vi "mav_connection_write.vi"(8 "error in":errorcluster, 9 "Connection Type":enum32{"TCP", "SERIAL", "UDP"}(tab), 10 "data in":string, 11 "mav_connection_in":T2) -> (0 "error out":errorcluster, 3 "mav_connection_out":T1)   [LabVIEW 2023]
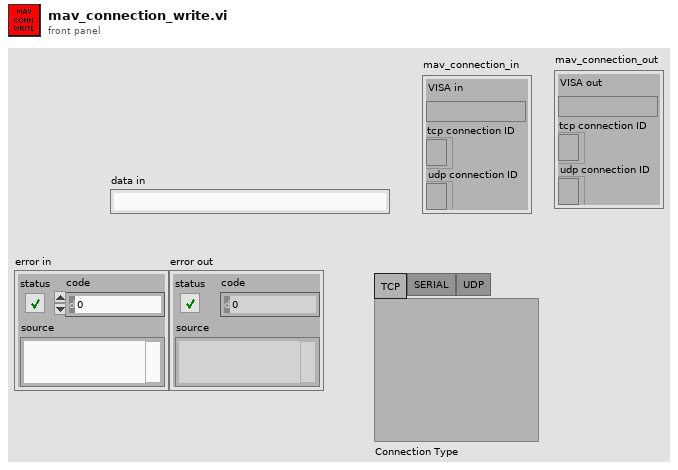
[diagram p1: front panel]
types:
  T1 = cluster{"VISA out":refnum<visa-resource-name>, "tcp connection ID":refnum<k5>, "udp connection ID":refnum<k16>}
  T2 = cluster{"VISA in":refnum<visa-resource-name>, "tcp connection ID":refnum<k5>, "udp connection ID":refnum<k16>}
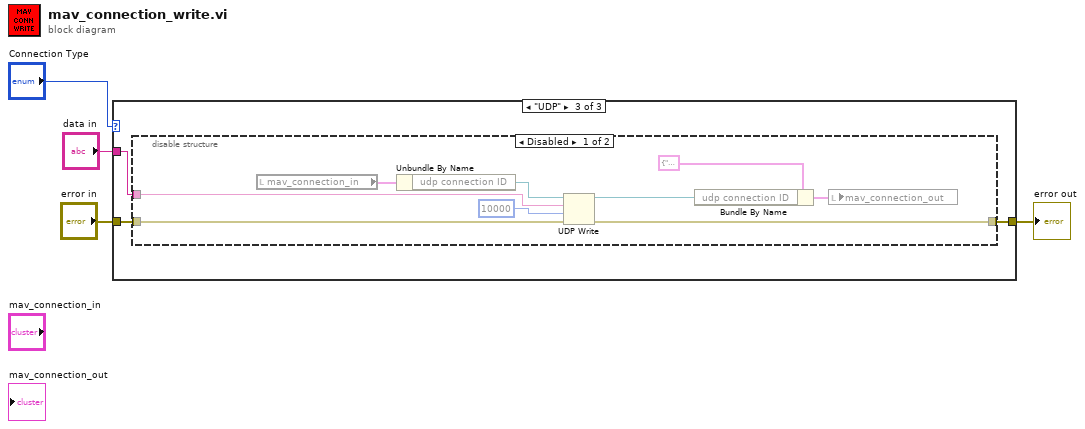
[diagram p0: block diagram]
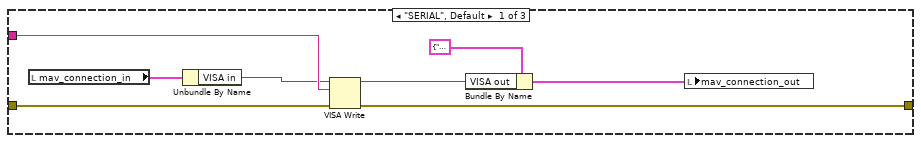
[diagram p2: hidden frame]
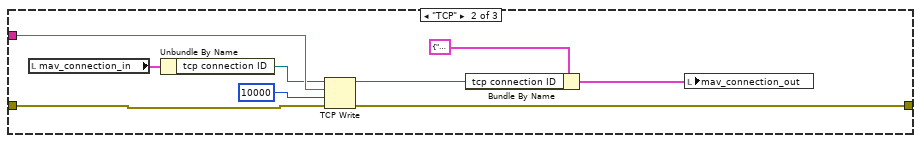
[diagram p3: hidden frame]
diagram:
  n1 = case shown="\"UDP\"" "Connection Type" {
    tunnel: "error in" -> [w12 w19 w24]
    tunnel: [w11 w20 w23] -> w3
    tunnel: "data in" -> [w10 w18 w22]
    frame "SERIAL", Default {
      n2 = local read "mav_connection_in"() -> (w7:T2)
      n3 = Unbundle By Name(w7) -> ("VISA in"=w6:refnum<visa-resource-name>)
      n4 = VISA Write(VISA resource name=w6, write buffer=w10, error in (no error)=w12) -> (VISA resource name out=w8:refnum<visa-resource-name>, error out=w11:errorcluster)  [unwired: 1 out]
      n5 = Bundle By Name(cluster=T1 {"VISA out"="", "tcp connection ID"=refnum, "udp connection ID"=refnum} ("mav_connection_out"), "VISA out"=w8) -> (w9:T1)
      n6 = local write "mav_connection_out"(w9) -> ()
    }
    frame "TCP" {
      n7 = local read "mav_connection_in"() -> (w17:T2)
      n8 = Unbundle By Name(w17) -> ("tcp connection ID"=w16:refnum<k5>)
      n9 = TCP Write(connection ID=w16, data in=w18, error in (no error)=w19, 9:10000 ("timeout ms (25000)")) -> (connection ID out=w14:refnum<k5>, error out=w20:errorcluster)  [unwired: 1 out]
      n10 = Bundle By Name(cluster=T1 {"VISA out"="", "tcp connection ID"=refnum, "udp connection ID"=refnum} ("mav_connection_out"), "tcp connection ID"=w14) -> (w15:T1)
      n11 = local write "mav_connection_out"(w15) -> ()
    }
    frame "UDP" {
      n12 = disable-structure shown="Disabled" {
        disable-tunnel: w24 -> [w27 _]
        disable-tunnel: [w26 _] -> w23
        disable-tunnel: w22 -> [w25 _]
        frame Disabled {
          n13 = local read "mav_connection_in"() -> (w30:T2)
          n14 = Unbundle By Name(w30) -> ("udp connection ID"=w31:refnum<k16>)
          n15 = UDP Write(connection ID=w31, data in=w25, 8:w27, 9:10000 ("timeout ms (25000)")) -> (error out=w26:errorcluster, 3:w33:refnum<k16>)  [unwired: 2 in]
          n16 = Bundle By Name(cluster=T1 {"VISA out"="", "tcp connection ID"=refnum, "udp connection ID"=refnum} ("mav_connection_out"), "udp connection ID"=w33) -> (w32:T1)
          n17 = local write "mav_connection_out"(w32) -> ()
        }
        frame Enabled {
        }
      }
    }
  }
  "error out" <- w3
